vi "Build Read Msg.vi"(4 "Address Areas":T2=132 items=["Input(I)"=129, "Output(Q)"=130, "Bit Memory(M)"=131, "Data(DB)"=132], 6 "#items":u16, 7 "Bit/Byte":u8(ring)=2 items=["Boolen"=1, "Byte"=2], 8 "error in (no error)":errorcluster, 9 "#offset":u32, 10 "# DB No.":u16, 11 "Siemens Ctr":T1) -> (0 "error out":errorcluster, 2 "Array Msg":u8[](array[numeric]) format="%.0x", 3 "Siemens Ctr out":T1)   [LabVIEW 2014, in "Simatic S7.lvlib"]
uses:
  Simatic S7.lvlib
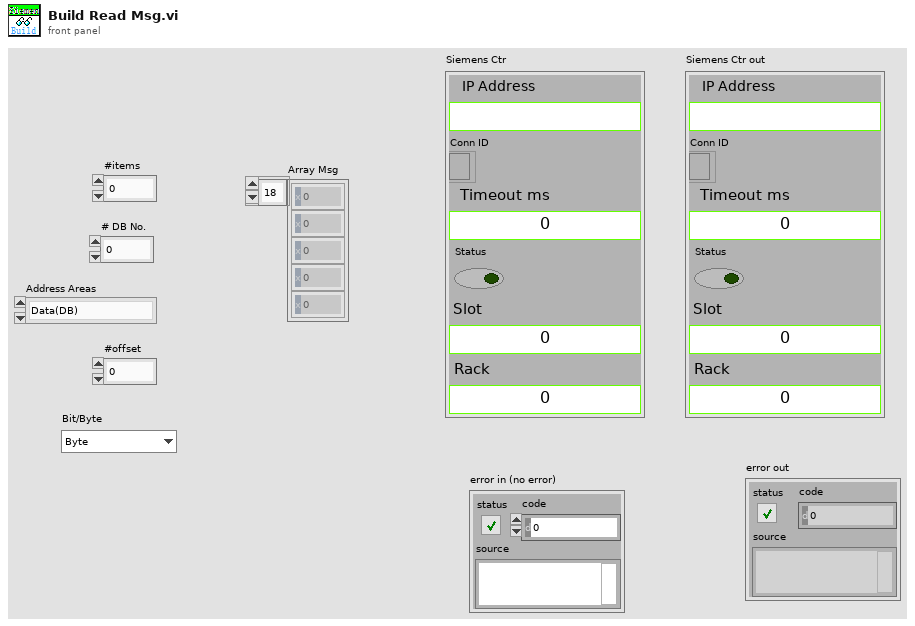
[diagram p1: front panel]
types:
  T1 = typedef "Simatic S7.lvlib/Siemens Ref.ctl" = cluster{"IP Address ":string, "Conn ID":refnum<k5>, "Timeout ms":i32, "Status":bool, "Slot":u16, "Rack":u16}
  T2 = typedef "Simatic S7.lvlib/Address Areas.ctl" = u8
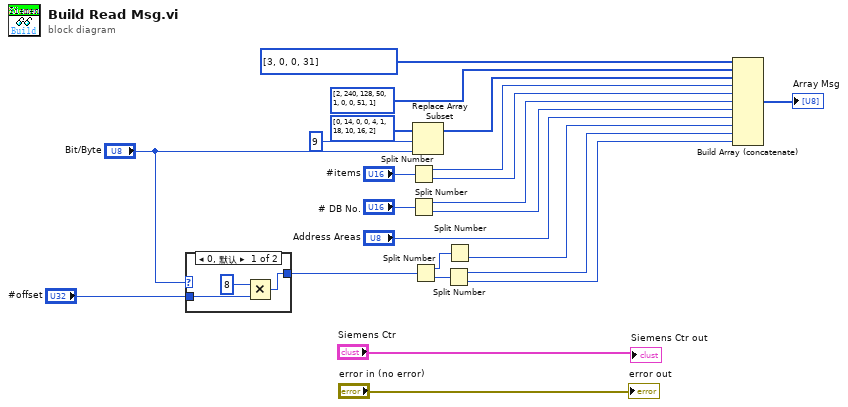
[diagram p0: block diagram]
diagram:
  n1 = case shown="0, 默认" "Bit/Byte" {
    tunnel: "#offset" -> [w25 w27]
    tunnel: [w26 w27] -> w1
    frame 0, Default {
      n2 = Multiply(x=u32 8, y=w25) -> (x*y=w26:u32)
    }
    frame 1 {
    }
  }
  n3 = Split Number(x="#items") -> (hi(x)=w19:u8, lo(x)=w18:u8)
  n4 = Split Number(x="# DB No.") -> (hi(x)=w16:u8, lo(x)=w15:u8)
  n5 = Split Number(x=w1) -> (hi(x)=w13:u16, lo(x)=w12:u16)
  n6 = Replace Array Subset(array=u8[] [0, 14, 0, 0, 4, 1, 18, 10, 16, 2], new element="Bit/Byte", index=9) -> (w5:u8[])
  n7 = Split Number(x=w12) -> (hi(x)=w10:u8, lo(x)=w9:u8)
  n8 = Split Number(x=w13) -> (lo(x)=w11:u8)  [unwired: 1 out]
  n9 = Build Array (concatenate)(u8[] [3, 0, 0, 31], u8[] [2, 240, 128, 50, 1, 0, 0, 51, 1], w5, w19, w18, w16, w15, "Address Areas", w11, w10, w9) -> (→"Array Msg":T2[])
  "error out" <- "error in (no error)"
  "Siemens Ctr out" <- "Siemens Ctr"
